vi "Stop.vi"(8 "error in (no error)":errorcluster, 10 "Message in":refnum<class "StopMessage.lvclass">, 11 "Cascade in":refnum<class "Cascade.lvclass">) -> (0 "error out":errorcluster, 3 "Cascade out":refnum<class "Cascade.lvclass">)   [LabVIEW 2012, in "Cascade.lvclass"]
doc: "This member function is called when the statemachine in the run.vi receives an 'stop' command. It relays the message to all observers of the component.\n\nOverride this member function in your derived class if you need additional stop functionality (but don't forget to call the parent method)."
uses:
  Cascade.lvclass
  <vilib>/Distrio/Murmex/StopMessage/StopMessage.lvclass
  <vilib>/Distrio/Murmex/Murmex/Murmex.lvclass
  Cascade.lvclass/Cascade.ctl
panel:
  # "This method is called when the STOP\ntrigger is sent. \n\nOverride this method when your component needs to\nrespond to this trigger. \n\nCall parent for proper implementation"
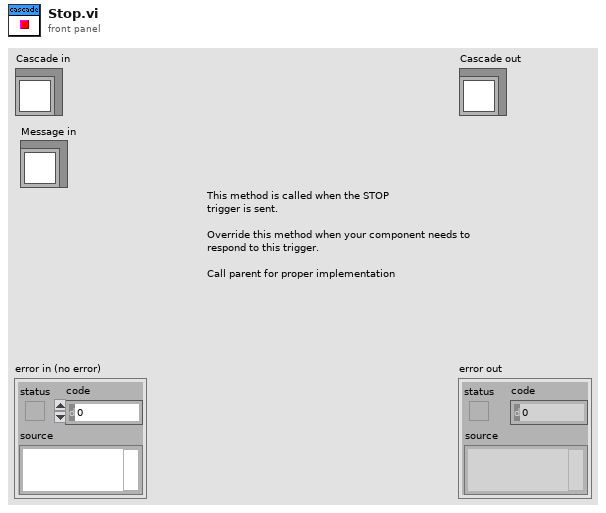
[diagram p1: front panel]
types:
  T1 = enum8{"Enabled", "Disabled", "Disabled and Grayed Out"}
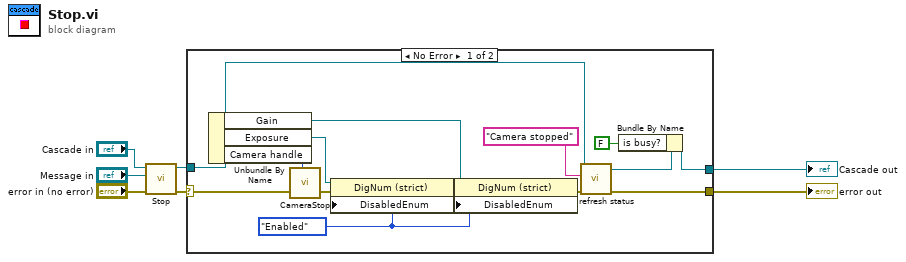
[diagram p0: block diagram]
diagram:
  n1 = call-parent "Stop.vi"("error in (no error)"="error in (no error)", "Message in"="Message in", "Murmex in"="Cascade in") -> ("error out"=w1:errorcluster, "Murmex out"=w2:refnum<class "Cascade.lvclass">)  [unwired: 7 in]
  n2 = case shown="No Error" w1 {
    selector: w1 -> [w20 w22]
    tunnel: w2 -> [w16 w23]
    tunnel: [w17 w22] -> w4
    tunnel: [w19 w23] -> w3
    frame No Error {
      w8 = T1."Enabled" ("Disabled")
      n3 = Unbundle By Name(w16) -> ("Gain"=w9:refnum<vi>, "Exposure"=w10:refnum<vi>, "Camera handle"=w21:u32)
      n4 = call <userlib>:"CameraStop.vi"("error in"=w20, "Camera Handle"=w21) -> ("error out"=w13:errorcluster)  [unwired: 1 out]
      n5 = property class="DigNum (strict)"(reference=w10, error in=w13, "DisabledEnum"=w8) -> (error out=w12:errorcluster)  [unwired: 1 out]
      n6 = property class="DigNum (strict)"(reference=w9, error in=w12, "DisabledEnum"=w8) -> (error out=w11:errorcluster)  [unwired: 1 out]
      n7 = call-dynamic "refresh status.vi"("error in (no error)"=w11, "String In"="Camera stopped", "Cascade in"=w16) -> ("error out"=w17:errorcluster, "Cascade out"=w15:refnum<class "Cascade.lvclass">)  [unwired: 7 in]
      n8 = Bundle By Name(cluster=w15, "is busy?"=FALSE ("runtime.is busy?")) -> (w19:refnum<class "Cascade.lvclass">)
    }
    frame Error {
    }
  }
  "error out" <- w4
  "Cascade out" <- w3
